vi "IP to Equipment.vi"(0 "RLT Equipment In":T2={"COM A"="COM3", "MW100"="MW100", "AG34970"="A-34972A", "COM B"="COM4", "COM C"="COM5", "COM D"="COM6"}, 2 "MW100 Semiphore":T3, 5 "Equipment In":T1={"COM Port"="COM3", "MW100"="MW100", "AG34970"="A-34972A", "Chamber"="WT500"}, 7 "Enable":bool, 11 "Error In":errorcluster) -> (4 "RLT Equip Out":T2, 6 "Equipment Out":T1={"COM Port"="COM3", "MW100"="MW100", "AG34970"="A-34972A", "Chamber"="WT500"}, 15 "Error Out":errorcluster)   [LabVIEW 2012]
uses:
  EquipReferences.ctl
  <vilib>/Utility/config.llb/Read Key (String).vi
  <vilib>/Utility/config.llb/Write Key (String).vi
  <vilib>/Utility/config.llb/NI_LVConfig.lvlib
panel:
  out "States":string[](array[string])
  in  "OK":bool
  in  "configuration file path":path=path "C:/work/flowconfig.ini"
  out "read buffer":string
  out "Error History":string[](array[string])
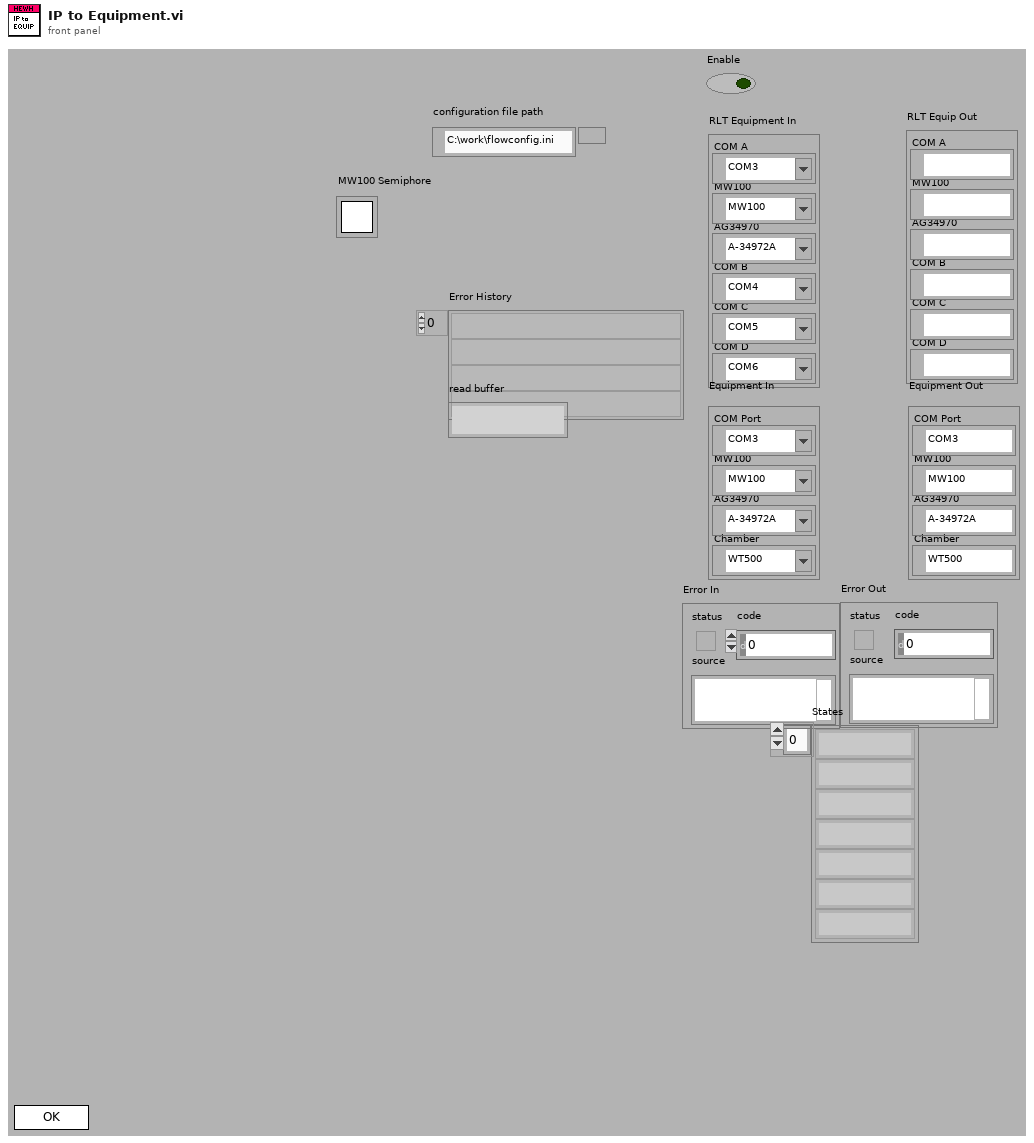
[diagram p1: front panel]
types:
  T1 = typedef "EquipReferences.ctl" = cluster{"COM Port":refnum<visa-resource-name>, "MW100":refnum<visa-resource-name>, "AG34970":refnum<visa-resource-name>, "Chamber":refnum<visa-resource-name>}
  T2 = cluster{"COM A":refnum<visa-resource-name>, "MW100":refnum<visa-resource-name>, "AG34970":refnum<visa-resource-name>, "COM B":refnum<visa-resource-name>, "COM C":refnum<visa-resource-name>, "COM D":refnum<visa-resource-name>}
  T3 = typedef "Semaphore RefNum" = refnum<k1>
  T4 = enum32{"invalid app kind", "Development System", "Run Time System", "Student Edition", "Embedded LabVIEW", "Evaluation", "Custom"}
  T5 = enum32{"Invalid", "Standard", "Closed", "Hidden", "Minimized", "Maximized"}
  T6 = cluster{"Core":cluster{"Current VI Reference":refnum<vi>, "Close Panel on Exit?":bool}, "Equipment In":T1, "RLT Equipment In":cluster{"COM A":refnum<visa-resource-name>, "MW100":refnum<visa-resource-name>, "AG34970":refnum<visa-resource-name>, "COM B":refnum<visa-resource-name>, "COM C":refnum<visa-resource-name>, "COM D":refnum<visa-resource-name>}, "configuration file path":path, "Error Flag":bool, "IP MW100":string, "IP A34972A":string, "semaphore":T3, "Local?":bool}
  T7 = cluster{"Current VI Reference":refnum<vi>, "Close Panel on Exit?":bool}
  T8 = typedef "NI_LVConfig.lvlib/Config Data RefNum.ctl" = refnum<k1>
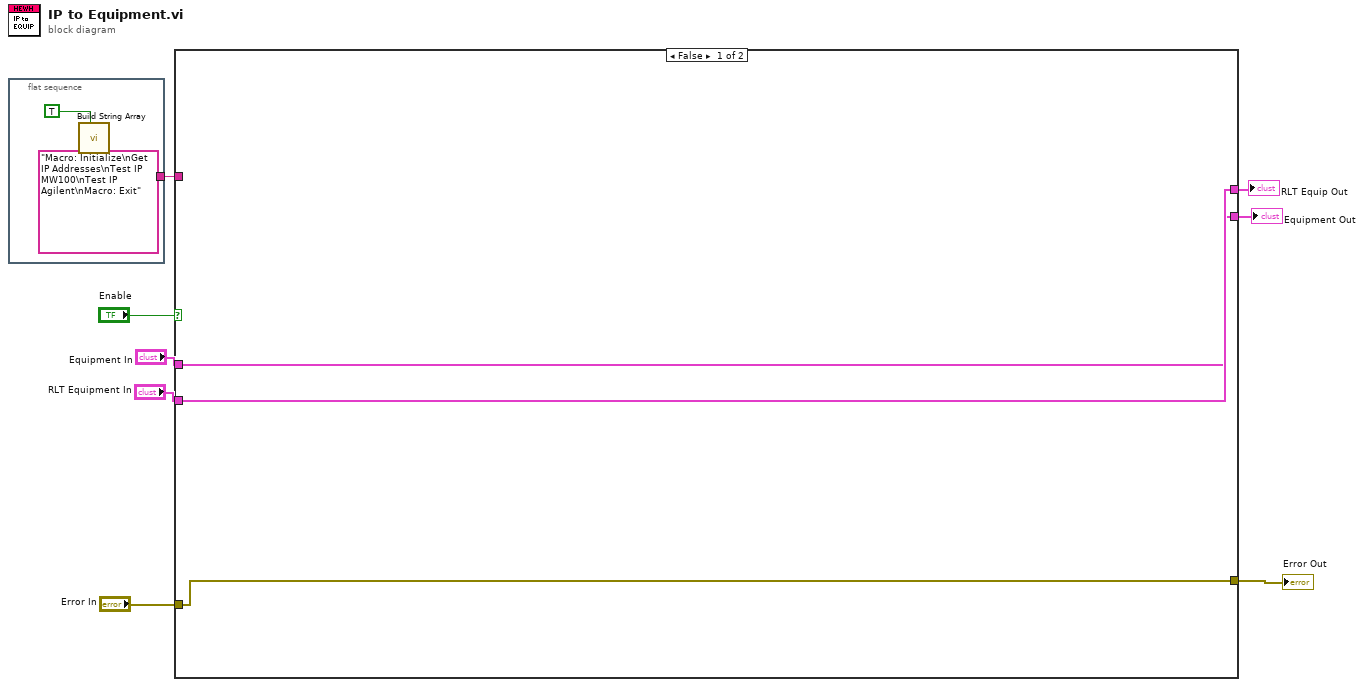
[diagram p0: block diagram]
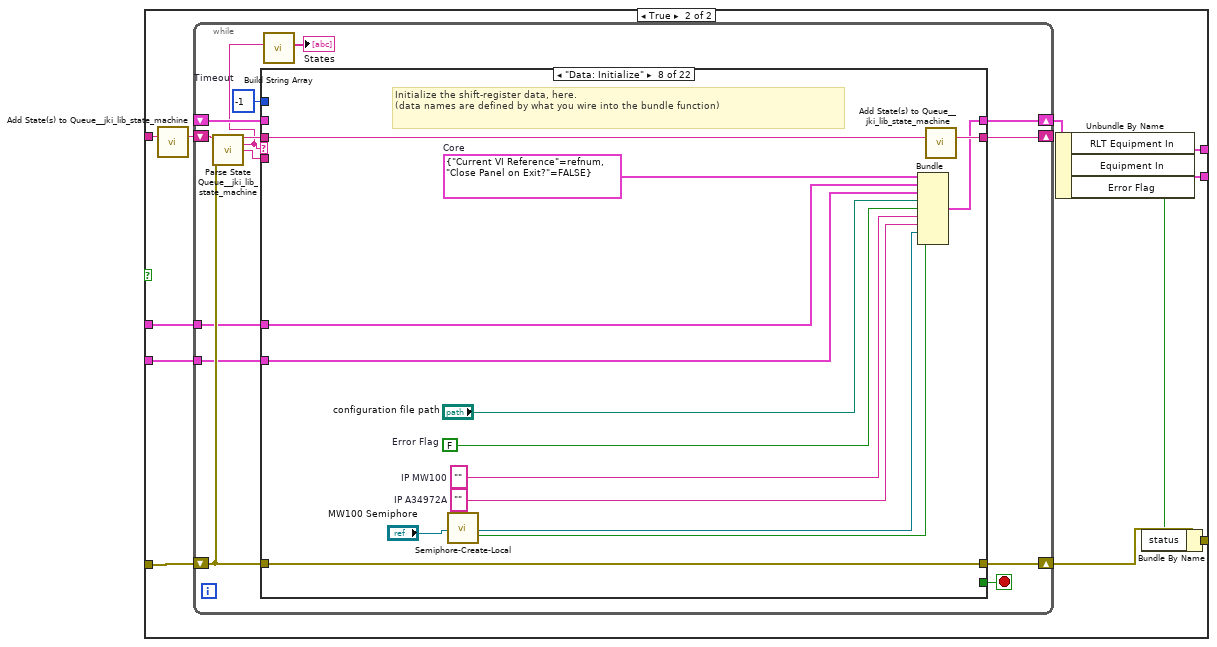
[diagram p2: hidden frame]
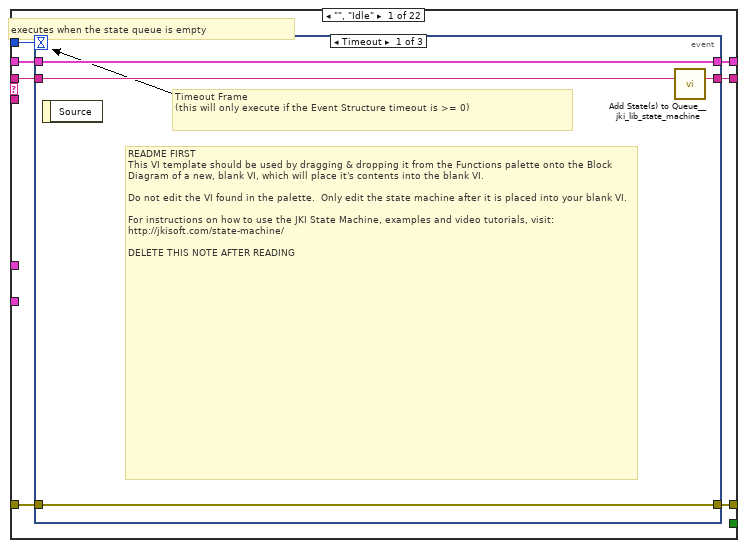
[diagram p3: hidden frame]
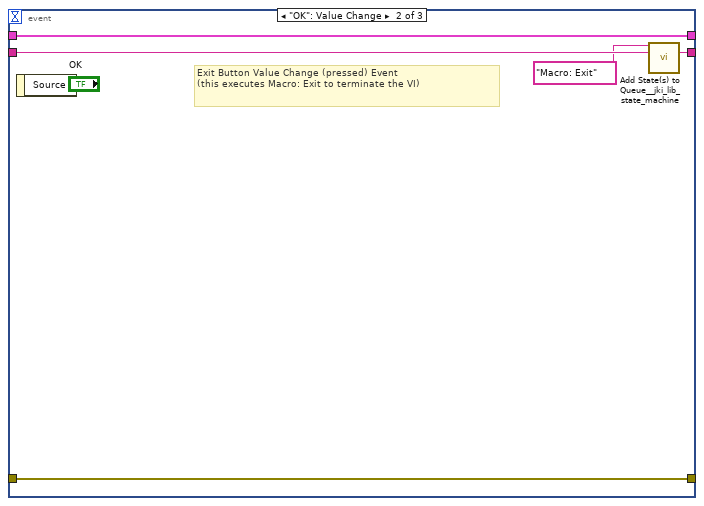
[diagram p4: hidden frame]
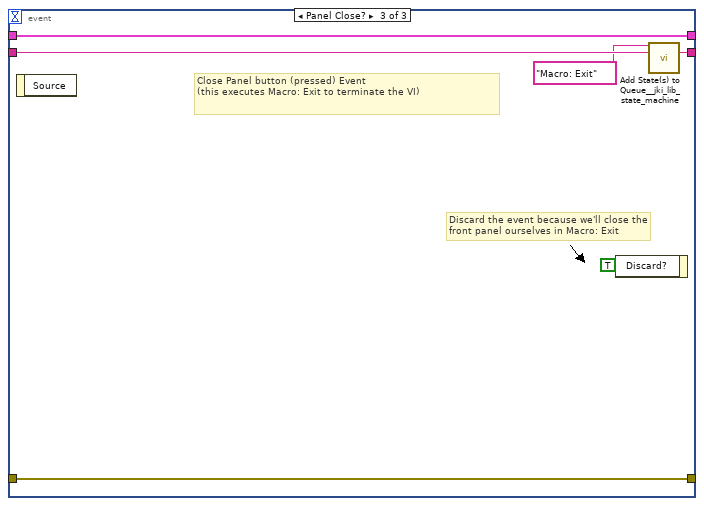
[diagram p5: hidden frame]
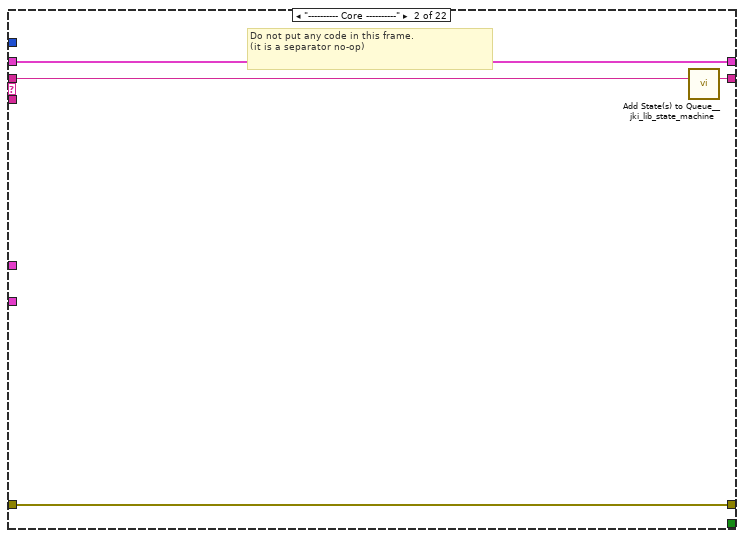
[diagram p6: hidden frame]
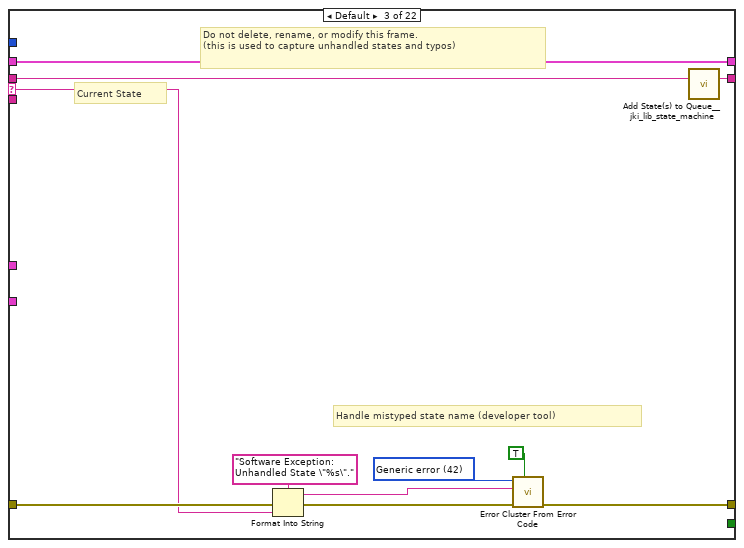
[diagram p7: hidden frame]
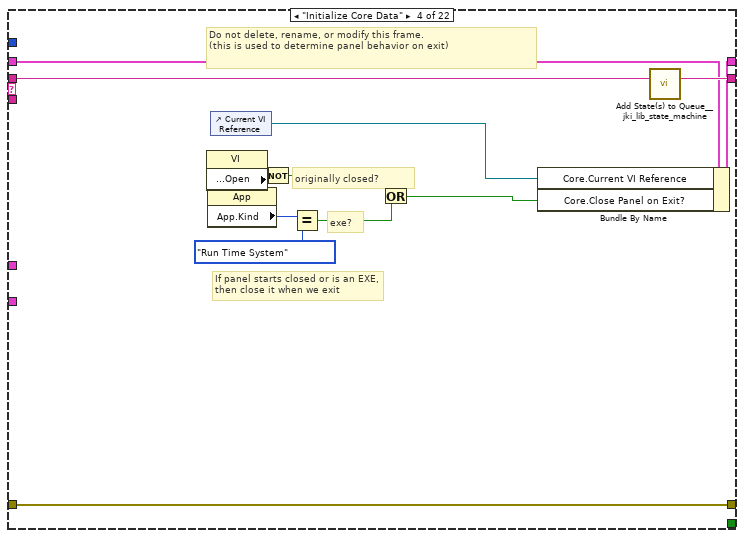
[diagram p8: hidden frame]
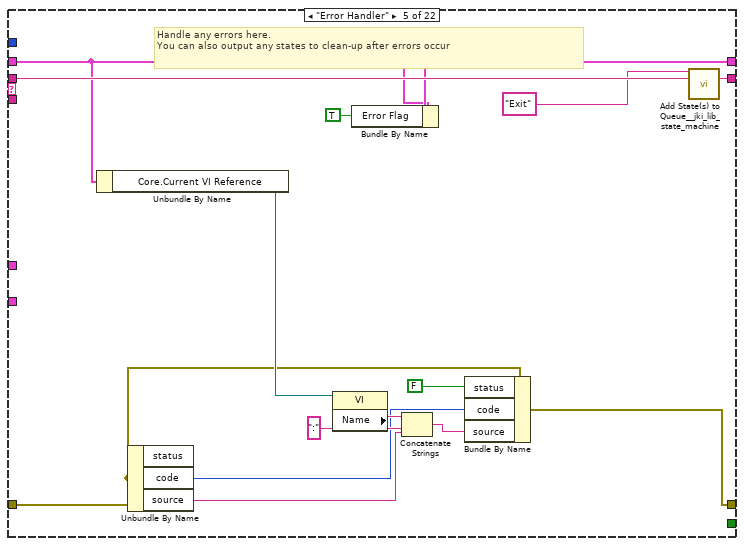
[diagram p9: hidden frame]
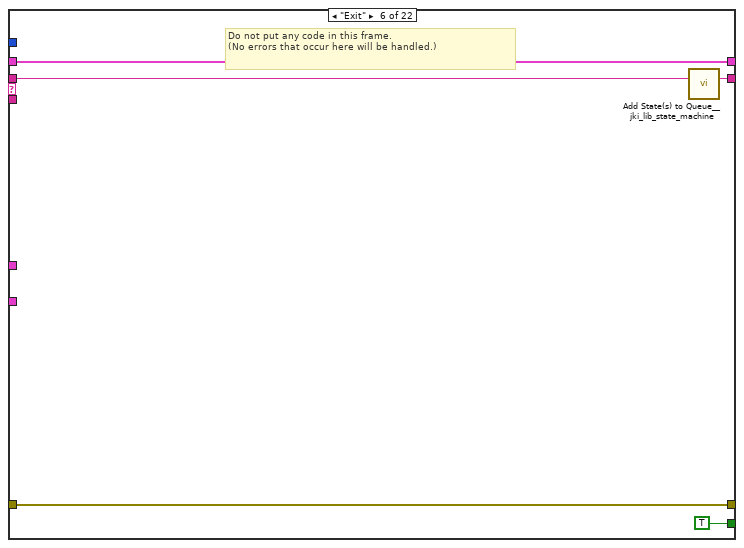
[diagram p10: hidden frame]
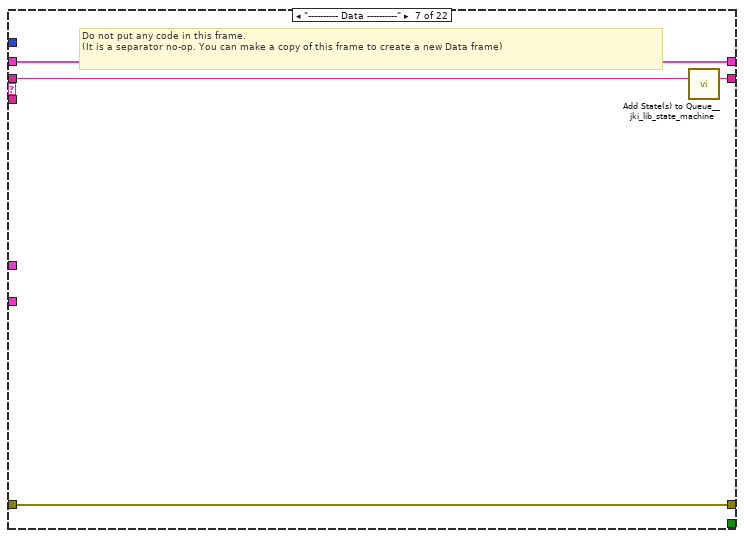
[diagram p11: hidden frame]
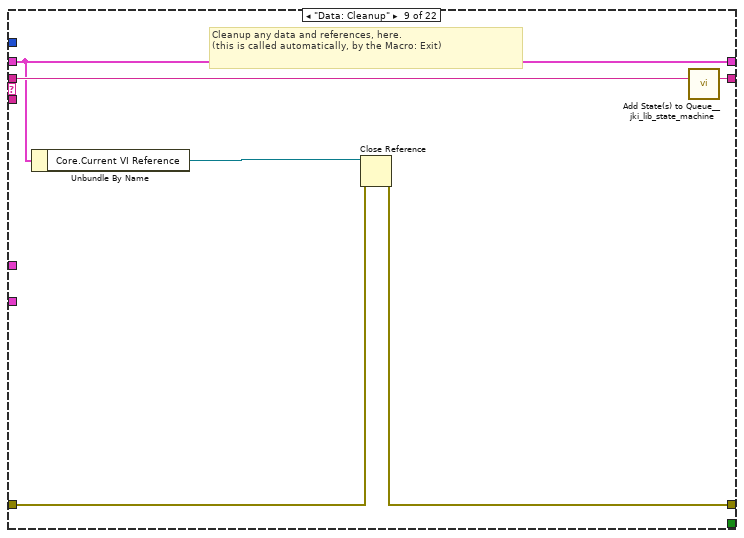
[diagram p12: hidden frame]
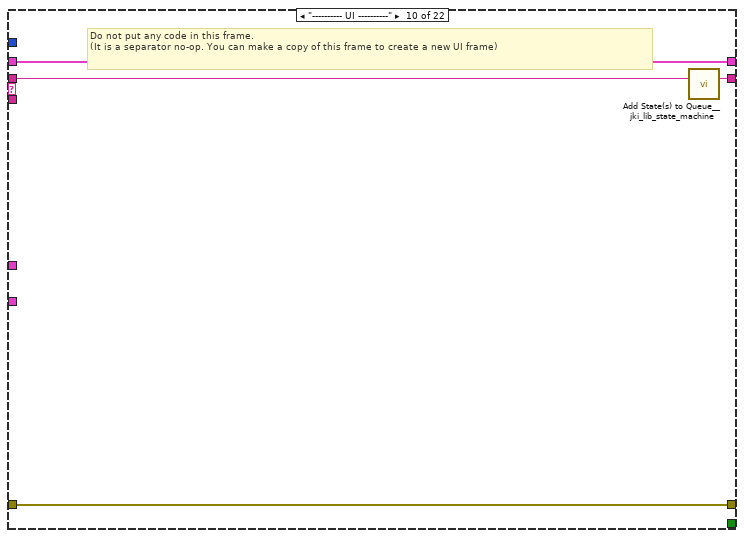
[diagram p13: hidden frame]
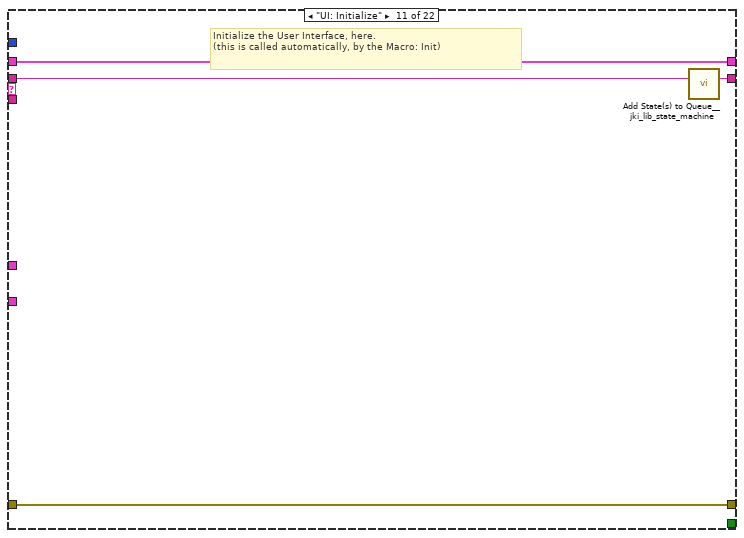
[diagram p14: hidden frame]
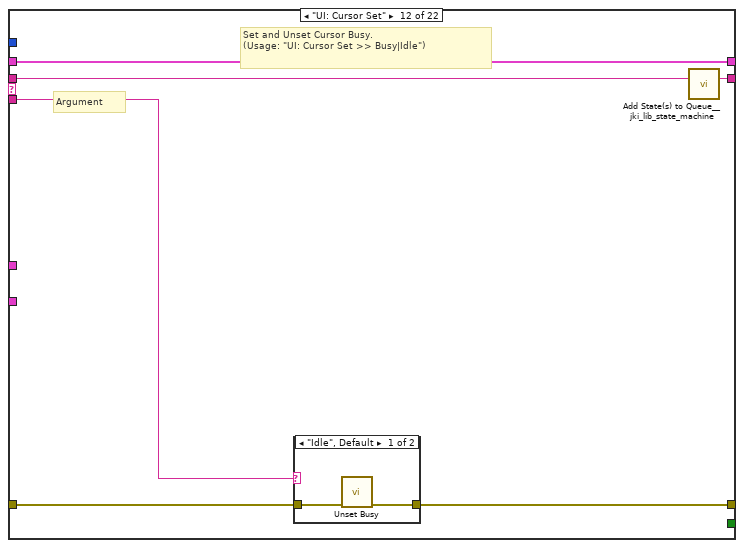
[diagram p15: hidden frame]
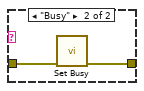
[diagram p16: hidden frame]
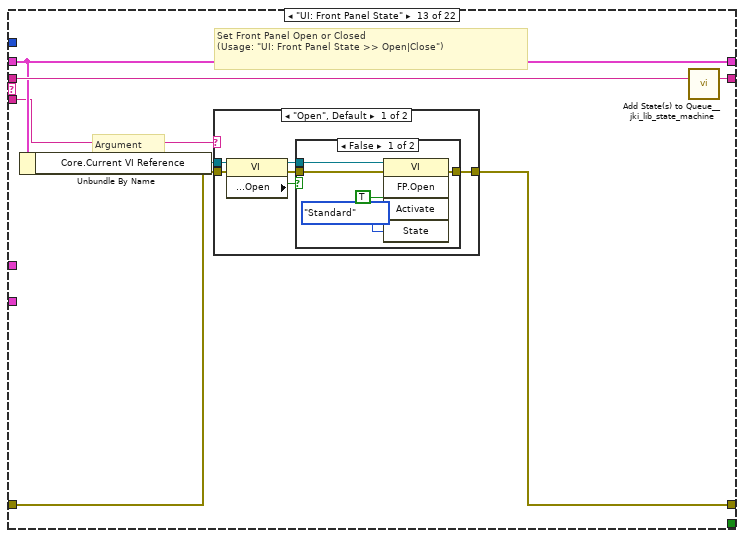
[diagram p17: hidden frame]
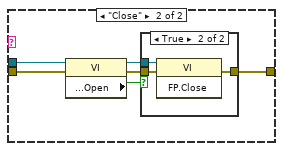
[diagram p19: hidden frame]
diagram:
  n1 = flat-sequence {
    tunnel: ["Macro: Initialize\nGet IP Addresses\nTest IP MW100\nTest IP Agilent\nMacro: Exit"] -> w8
    frame #0 {
      n2 = call "Build String Array.vi"("Initialize"=TRUE) -> ()  [unwired: 10 in, 1 out]
    }
  }
  n3 = case shown="False" "Enable" {
    tunnel: w8 -> [_ w23]
    tunnel: "Error In" -> [w11 w22]
    tunnel: [w11 w20] -> w6
    tunnel: [w13 w17] -> w5
    tunnel: [w12 w16] -> w4
    tunnel: "Equipment In" -> [w12 w15]
    tunnel: "RLT Equipment In" -> [w13 w14]
    frame False {
    }
    frame True {
      n4 = call <vilib>:"Add State(s) to Queue__jki_lib_state_machine.vi"("State(s) in (\"\")"=w23) -> ("States Out"=w24:string)  [unwired: 14 in]
      n5 = while {
        shift-right: [w32] -> w21
        shift-left: _ -> [w31]
        shift-right: [w35] -> w19
        shift-left: w22 -> [w29]
        shift-right: [w34] -> _
        shift-left: w24 -> [w36]
        tunnel: w15 -> [w26]
        tunnel: w14 -> [w25]
        stop <- w33 stop-if-true
        w30 = -1  # Timeout
        n6 = call <vilib>:"Parse State Queue__jki_lib_state_machine.vi"("State Queue"=w36, "Error In (no error)"=w29) -> ("Remaining States"=w38:string, "Current State"=w27:string, "Arguments"=w37:string)  [unwired: 11 in]
        n7 = case shown="\"Data: Initialize\"" w27 {
          selector: w27 -> [_ _ w65 _ _ _ _ _ _ _ _ _ _ _ _ _ _ _ _ _ _ _]
          tunnel: w38 -> [w45 w64 w69 w87 w102 w107 w111 w125 w131 w135 w139 w145 w156 w182 w187 w200 w204 w227 w238 w259 w272 w293]
          tunnel: w37 -> [_ _ _ _ _ _ _ _ _ _ _ w140 w150 _ _ _ _ _ _ _ _ _]
          tunnel: w31 -> [w43 w61 w67 w78 w93 w103 w108 _ w126 w132 w137 w143 w152 w179 w184 w190 w201 w215 w235 w242 w262 w287]
          tunnel: [w42 w62 w71 w84 w89 w105 w109 w122 w127 w133 w136 w141 w153 w180 w185 w188 w202 w205 w236 w246 w270 w291] -> w35
          tunnel: w29 -> [w41 w62 w70 w84 w88 w105 w109 w122 w128 w133 w136 w142 w154 w180 w185 w189 w202 w220 w236 w256 w270 w291]
          tunnel: [w44 w63 w68 w86 w101 w106 w110 w124 w130 w134 w138 w144 w155 w181 w186 w199 w203 w226 w237 w258 w271 w292] -> w34
          tunnel: [_ _ _ _ _ TRUE _ _ _ _ _ _ _ _ _ _ _ _ _ _ _ _] -> w33
          tunnel: [w40 w61 w67 w85 w99 w103 w108 w123 w126 w132 w137 w143 w152 w179 w184 w190 w201 w214 w235 w243 w261 w286] -> w32
          tunnel: w30 -> [w39 _ _ _ _ _ _ _ _ _ _ _ _ _ _ _ _ _ _ _ _ _]
          tunnel: w26 -> [_ _ _ _ _ _ _ w113 _ _ _ _ _ _ _ _ _ _ _ _ _ _]
          tunnel: w25 -> [_ _ _ _ _ _ _ w112 _ _ _ _ _ _ _ _ _ _ _ _ _ _]
          frame "", "Idle" {
            # "executes when the state queue is empty"
            n8 = event shown="[0] Timeout" {
              selector: _ -> [_ _ _]
              dyn-events: _ -> [_ _ _]
              timeout: w39 -> [_ _ _]
              tunnel: w45 -> [w49 w54 w60]
              tunnel: [w48 w53 w59] -> w44
              tunnel: w43 -> [w46 w51 w57]
              tunnel: [w47 w52 w58] -> w42
              tunnel: w41 -> [w47 w52 w58]
              tunnel: [w46 w51 w57] -> w40
              event Timeout {
                # "README FIRST\nThis VI template should be used by dragging & dropping it from the Functions palette onto the Block Diagram of a new, blank VI, which will place it's contents into the blank VI.\n\nDo not edit the VI found in the palette.  Only edit the state machine after it is placed into your blank VI.\n\nFor instructions on how to use the JKI State Machine, examples and video tutorials, visit:\nhttp://jkisoft.com/state-machine/\n\nDELETE THIS NOTE AFTER READING"
                # "Timeout Frame\n(this will only execute if the Event Structure timeout is >= 0)"
                n9 = event-data() -> ()  [unwired: 1 in, 1 out]
                n10 = call <vilib>:"Add State(s) to Queue__jki_lib_state_machine.vi"("State(s) in (\"\")"=w49) -> ("States Out"=w48:string)  [unwired: 14 in]
              }
              event "OK": Value Change {
                # "Exit Button Value Change (pressed) Event\n(this executes Macro: Exit to terminate the VI)"
                n11 = event-data() -> ()  [unwired: 1 in, 1 out]
                n12 = call <vilib>:"Add State(s) to Queue__jki_lib_state_machine.vi"("State(s) in Front (\"\")"="Macro: Exit", "State(s) in (\"\")"=w54) -> ("States Out"=w53:string)  [unwired: 13 in]
              }
              event Panel Close? {
                # "Discard the event because we'll close the front panel ourselves in Macro: Exit"
                # "Close Panel button (pressed) Event\n(this executes Macro: Exit to terminate the VI)"
                n13 = event-data() -> ()  [unwired: 1 in, 1 out]
                n14 = event-data("Discard?"=TRUE) -> ()  [unwired: 1 in, 1 out]
                n15 = call <vilib>:"Add State(s) to Queue__jki_lib_state_machine.vi"("State(s) in Front (\"\")"="Macro: Exit", "State(s) in (\"\")"=w60) -> ("States Out"=w59:string)  [unwired: 13 in]
              }
            }
          }
          frame "---------- Core ----------" {
            # "Do not put any code in this frame.\n(it is a separator no-op)"
            n16 = call <vilib>:"Add State(s) to Queue__jki_lib_state_machine.vi"("State(s) in (\"\")"=w64) -> ("States Out"=w63:string)  [unwired: 14 in]
          }
          frame Default {
            w74 = 42 items=["No error", "Argument error", "Memory is full", "Out of zone", "End of file", "File already open", "Generic file I/O error", "File not found", "File permission error", "Disk is full", "Duplicate path", "Too many files open", "System feature not enabled", "Resource file not found", "Cannot add resource", "Resource not found", "Image not found", "Image memory error", "Pen does not exist", "Config type invalid", "Config token not found", "Config parse error", "Config memory error", "Bad external code format", "Bad external code offset", "External code not present", "Null window", "Destroy window error", "Null menu", "Print aborted", "Bad print record", "Print driver error", "Windows error during printing", "Memory error during printing", "Print dialog error", "Generic print error", "Invalid device refnum", "Device not found", "Device parameter error", "Device unit error", "Cannot open device", "Device call aborted", "Generic error", "Cancelled by user", "Object ID too low", "Object ID too high", "Object not in heap", "Unknown heap", "Unknown object (invalid DefProc)", "Unknown object (DefProc not in table)", "Message out of range", "Invalid (null) method", "Unknown message", "Manager call not supported", "Bad address", "Network operation in progress", "Network operation timed out", "Connection is busy", "Network attribute not supported", "Network error", "Address in use", "System out of memory", "Connection aborted", "Connection refused", "Not connected", "Already connected", "Connection closed", "Initialization error (interapplication manager)", "Bad occurrence", "Wait on unbound occurrence handler", "Occurrence queue overflow", "Datalog type conflict", "Unused", "Unrecognized type (interapplication manager)", "Memory corrupt", "Failed to make temporary DLL", "Old CIN version", "Drag socket not found", "Failed to load drop-object", "Failed to register OLE object", "Failed to release OLE object", "Format specifier type mismatch", "Unknown format specifier", "Too few format specifiers", "Too many format specifiers", "Scan failed", "Newer CIN version", "Error converting to variant", "Runtime menu error", "Password tampered", "Variant attribute not found", "Incompatible variant data type", "Event data is not available", "Event Store is not present", "Occurrence is not found", "Event Queue is not created", "Event info is not available", "Refnum passed is NULL", "Error retrieving Class GUID", "Error retrieving CoClass GUID", "Error retrieving TypeLib GUID.", "Bad built application magic bytes.", "Specific driver is different from the specific driver associated with the Logical Name.", "There is no session opened to the class driver.", "Max Error", "MAX - Error with config objects", "MAX - Error loading configuration", "MAX - Group not supported"]
            # "Current State"
            # "Do not delete, rename, or modify this frame.\n(this is used to capture unhandled states and typos)"
            # "Handle mistyped state name (developer tool)"
            n17 = Format Into String(format string="Software Exception: Unhandled State \"%s\"." ("message"), error in=w70, w65) -> (resulting string=w73:string, error out=w72:errorcluster)  [unwired: 1 in]
            n18 = call <vilib>:"Error Cluster From Error Code.vi"("show call chain? (False)"=TRUE, "error in (no error)"=w72, "error message (\"\")"=w73, "error code (0)"=w74) -> ("error out"=w71:errorcluster)  [unwired: 5 in]
            n19 = call <vilib>:"Add State(s) to Queue__jki_lib_state_machine.vi"("State(s) in (\"\")"=w69) -> ("States Out"=w68:string)  [unwired: 14 in]
          }
          frame "Initialize Core Data" {
            # "Do not delete, rename, or modify this frame.\n(this is used to determine panel behavior on exit)"
            # "originally closed?"
            # "exe?"
            # "If panel starts closed or is an EXE, then close it when we exit"
            n20 = property class="VI"() -> ("Front Panel.Open"=w83:bool)  [unwired: 2 in, 2 out]
            n21 = property class="App"() -> ("App.Kind"=w82:T4)  [unwired: 2 in, 2 out]
            n22 = control-ref of="Current VI Reference"() -> (w76:refnum<vi>)
            n23 = Not(x=w83) -> (.not. x?=w80:bool)
            n24 = Equal?(x=w82, y=T4."Run Time System" ("Application:Kind")) -> (x = y?=w79:bool)
            n25 = Or(x=w80, y=w79) -> (x .or. y?=w77:bool)
            n26 = Bundle By Name(cluster=w78, "Core.Current VI Reference"=w76, "Core.Close Panel on Exit?"=w77) -> (w85:T6)
            n27 = call <vilib>:"Add State(s) to Queue__jki_lib_state_machine.vi"("State(s) in (\"\")"=w87) -> ("States Out"=w86:string)  [unwired: 14 in]
          }
          frame "Error Handler" {
            # "Handle any errors here.\nYou can also output any states to clean-up after errors occur"
            n28 = Unbundle By Name(w93) -> ("Core.Current VI Reference"=w92:refnum<vi>)
            n29 = Unbundle By Name(w88) -> ("code"=w91:i32, "source"=w90:string)  [unwired: 1 out]
            n30 = property class="VI"(reference=w92) -> ("Name"=w94:string)  [unwired: 1 in, 2 out]
            n31 = Bundle By Name(cluster=w93, "Error Flag"=TRUE) -> (w99:T6)
            n32 = Concatenate Strings(w94, ":" ("string"), w90) -> (w96:string)
            n33 = Bundle By Name(cluster=w88, "status"=FALSE, "code"=w91, "source"=w96) -> (w89:errorcluster)
            n34 = call <vilib>:"Add State(s) to Queue__jki_lib_state_machine.vi"("State(s) in Front (\"\")"="Exit", "State(s) in (\"\")"=w102) -> ("States Out"=w101:string)  [unwired: 13 in]
          }
          frame "Exit" {
            # "Do not put any code in this frame.\n(No errors that occur here will be handled.)"
            n35 = call <vilib>:"Add State(s) to Queue__jki_lib_state_machine.vi"("State(s) in (\"\")"=w107) -> ("States Out"=w106:string)  [unwired: 14 in]
          }
          frame "---------- Data ----------" {
            # "Do not put any code in this frame.\n(It is a separator no-op. You can make a copy of this frame to create a new Data frame)"
            n36 = call <vilib>:"Add State(s) to Queue__jki_lib_state_machine.vi"("State(s) in (\"\")"=w111) -> ("States Out"=w110:string)  [unwired: 14 in]
          }
          frame "Data: Initialize" {
            w116 = ""  # IP A34972A
            w117 = ""  # IP MW100
            w118 = FALSE  # Error Flag
            w121 = T7 {"Current VI Reference"=refnum, "Close Panel on Exit?"=FALSE}  # Core
            # "Initialize the shift-register data, here.\n(data names are defined by what you wire into the bundle function)"
            n37 = call "Semiphore-Create-Local.vi"("Semiphore"="MW100 Semiphore") -> ("semaphore"=w115:T3, "Local?"=w114:bool)  [unwired: 16 in, 1 out]
            n38 = Bundle("Core"=w121, "Equipment In"=w113, "RLT Equipment In"=w112, "configuration file path"="configuration file path", "Error Flag"=w118, "IP MW100"=w117, "IP A34972A"=w116, "semaphore"=w115, "Local?"=w114) -> (w123:T6)  [unwired: 1 in]
            n39 = call <vilib>:"Add State(s) to Queue__jki_lib_state_machine.vi"("State(s) in (\"\")"=w125) -> ("States Out"=w124:string)  [unwired: 14 in]
          }
          frame "Data: Cleanup" {
            # "Cleanup any data and references, here.\n(this is called automatically, by the Macro: Exit)"
            n40 = Unbundle By Name(w126) -> ("Core.Current VI Reference"=w129:refnum<vi>)
            n41 = Close Reference(reference=w129, error in (no error)=w128) -> (error out=w127:errorcluster)
            n42 = call <vilib>:"Add State(s) to Queue__jki_lib_state_machine.vi"("State(s) in (\"\")"=w131) -> ("States Out"=w130:string)  [unwired: 14 in]
          }
          frame "---------- UI ----------" {
            # "Do not put any code in this frame.\n(It is a separator no-op. You can make a copy of this frame to create a new UI frame)"
            n43 = call <vilib>:"Add State(s) to Queue__jki_lib_state_machine.vi"("State(s) in (\"\")"=w135) -> ("States Out"=w134:string)  [unwired: 14 in]
          }
          frame "UI: Initialize" {
            # "Initialize the User Interface, here.\n(this is called automatically, by the Macro: Init)"
            n44 = call <vilib>:"Add State(s) to Queue__jki_lib_state_machine.vi"("State(s) in (\"\")"=w139) -> ("States Out"=w138:string)  [unwired: 14 in]
          }
          frame "UI: Cursor Set" {
            # "Argument"
            # "Set and Unset Cursor Busy.\n(Usage: \"UI: Cursor Set >> Busy|Idle\")"
            n45 = case shown="\"Idle\", Default" w140 {
              tunnel: w142 -> [w147 w149]
              tunnel: [w146 w148] -> w141
              frame "Idle", Default {
                n46 = call <vilib>:"Unset Busy.vi"("error in (no error)"=w147) -> ("error out"=w146:errorcluster)  [unwired: 10 in]
              }
              frame "Busy" {
                n47 = call <vilib>:"Set Busy.vi"("error in (no error)"=w149) -> ("error out"=w148:errorcluster)  [unwired: 9 in, 1 out]
              }
            }
            n48 = call <vilib>:"Add State(s) to Queue__jki_lib_state_machine.vi"("State(s) in (\"\")"=w145) -> ("States Out"=w144:string)  [unwired: 14 in]
          }
          frame "UI: Front Panel State" {
            # "Argument"
            # "Set Front Panel Open or Closed\n(Usage: \"UI: Front Panel State >> Open|Close\")"
            n49 = Unbundle By Name(w152) -> ("Core.Current VI Reference"=w151:refnum<vi>)
            n50 = case shown="\"Open\", Default" w150 {
              tunnel: w154 -> [w160 w173]
              tunnel: [w162 w174] -> w153
              tunnel: w151 -> [w161 w171]
              frame "Open", Default {
                n51 = property class="VI"(reference=w161, error in=w160) -> (reference out=w158:refnum<vi>, error out=w159:errorcluster, "Front Panel.Open"=w157:bool)
                n52 = case shown="False" w157 {
                  tunnel: [w165 w168] -> w162
                  tunnel: w159 -> [w164 w168]
                  tunnel: w158 -> [w163 _]
                  frame False {
                    n53 = invoke class="VI" method="FP.Open"(reference=w163, error in=w164, "Activate"=TRUE, "State"=T5."Standard") -> (error out=w165:errorcluster)  [unwired: 1 in, 4 out]
                  }
                  frame True {
                  }
                }
              }
              frame "Close" {
                n54 = property class="VI"(reference=w171, error in=w173) -> (reference out=w170:refnum<vi>, error out=w172:errorcluster, "Front Panel.Open"=w169:bool)
                n55 = case shown="True" w169 {
                  tunnel: [w175 w178] -> w174
                  tunnel: w172 -> [w175 w177]
                  tunnel: w170 -> [_ w176]
                  frame False {
                  }
                  frame True {
                    n56 = invoke class="VI" method="FP.Close"(reference=w176, error in=w177) -> (error out=w178:errorcluster)  [unwired: 1 in, 2 out]
                  }
                }
              }
            }
            n57 = call <vilib>:"Add State(s) to Queue__jki_lib_state_machine.vi"("State(s) in (\"\")"=w156) -> ("States Out"=w155:string)  [unwired: 14 in]
          }
          frame "---------- Macro ----------" {
            # "Do not put any code in this frame.\n(It is a separator no-op. You can make a copy of this frame to create a new Macro frame)"
            n58 = call <vilib>:"Add State(s) to Queue__jki_lib_state_machine.vi"("State(s) in (\"\")"=w182) -> ("States Out"=w181:string)  [unwired: 14 in]
          }
          frame "Macro: Initialize" {
            # "Initialization Macro\n(This is called once, when the VI starts)"
            n59 = call <vilib>:"Add State(s) to Queue__jki_lib_state_machine.vi"("State(s) in Front (\"\")"="Data: Initialize\nInitialize Core Data", "State(s) in (\"\")"=w187) -> ("States Out"=w186:string)  [unwired: 13 in]
          }
          frame "Macro: Exit" {
            # "Exit Macro\n(This is called once, when the VI exits)"
            n60 = Unbundle By Name(w190) -> ("Core.Close Panel on Exit?"=w198:bool)
            n61 = Unbundle By Name(w190) -> ("semaphore"=w192:T3, "Local?"=w191:bool)
            n62 = call "Semiphore-Destroy-Local.vi"("Semiphore"=w192, "Local?"=w191, "error in (no error)"=w189) -> ("error out"=w188:errorcluster)  [unwired: 16 in]
            n63 = Select(t="UI: Front Panel State >> Close", s=w198, f="") -> (s? t:f=w195:string)
            n64 = call <vilib>:"Add State(s) to Queue__jki_lib_state_machine.vi"("State(s) in (\"\")"=w195, "State(s) at Back (\"\")"="Data: Cleanup\nExit") -> ("States Out"=w193:string)  [unwired: 13 in]
            n65 = call <vilib>:"Add State(s) to Queue__jki_lib_state_machine.vi"("State(s) in Front (\"\")"=w193, "State(s) in (\"\")"=w200) -> ("States Out"=w199:string)  [unwired: 13 in]
          }
          frame "---------- New Category ----------" {
            # "Template Separator\n(You can make a copy of, or modify, this frame)"
            n66 = call <vilib>:"Add State(s) to Queue__jki_lib_state_machine.vi"("State(s) in (\"\")"=w204) -> ("States Out"=w203:string)  [unwired: 14 in]
          }
          frame "Get IP Addresses" {
            w222 = "IP Addresses" ("section")
            n67 = Unbundle By Name(w215) -> ("configuration file path"=w218:path)
            n68 = call <vilib>:"Open Config Data.vi"("error in (no error)"=w220, "create file if necessary (T)"=FALSE, "configuration file path"=w218) -> ("error out"=w221:errorcluster, "refnum"=w223:T8)  [unwired: 6 in, 1 out]
            n69 = call-poly <vilib>:"Read Key.vi"("section"=w222, "error in (no error)"=w221, "key"="IP MW100", "refnum"=w223) -> ("error out"=w225:errorcluster, "value"=w213:string, "found?"=w209:bool, "refnum out"=w224:T8)  [unwired: 4 in]
            n70 = call-poly <vilib>:"Read Key.vi"("section"=w222, "error in (no error)"=w225, "key"="IP A34972A", "refnum"=w224) -> ("error out"=w206:errorcluster, "value"=w212:string, "found?"=w210:bool, "refnum out"=w207:T8)  [unwired: 4 in]
            n71 = call <vilib>:"Close Config Data.vi"("error in (no error)"=w206, "refnum"=w207) -> ("error out"=w205:errorcluster)  [unwired: 8 in, 1 out]
            n72 = And(x=w210, y=w209) -> (x .and. y?=w211:bool)
            n73 = case shown="True" w211 {
              tunnel: w215 -> [w229 w234]
              tunnel: [w229 w233] -> w214
              tunnel: w213 -> [_ w232]
              tunnel: w212 -> [_ w231]
              tunnel: ["Prompt for IP" ("State(s) in Front (\"\")") "" ("State(s) in Front (\"\")")] -> w208
              frame False {
              }
              frame True {
                n74 = Bundle By Name(cluster=w234, "IP MW100"=w232, "IP A34972A"=w231) -> (w233:T6)
              }
            }
            n75 = call <vilib>:"Add State(s) to Queue__jki_lib_state_machine.vi"("State(s) in Front (\"\")"=w208, "State(s) in (\"\")"=w227) -> ("States Out"=w226:string)  [unwired: 13 in]
          }
          frame "Merge IP Addresses" {
            n76 = call <vilib>:"Add State(s) to Queue__jki_lib_state_machine.vi"("State(s) in (\"\")"=w238) -> ("States Out"=w237:string)  [unwired: 14 in]
          }
          frame "Prompt for IP" {
            w252 = "IP Addresses" ("section")
            n77 = Unbundle By Name(w242) -> ("configuration file path"=w241:path, "IP MW100"=w240:string, "IP A34972A"=w239:string)
            n78 = call <vilib>:"Open Config Data.vi"("error in (no error)"=w256, "create file if necessary (T)"=FALSE, "configuration file path"=w241) -> ("error out"=w255:errorcluster, "refnum"=w249:T8)  [unwired: 6 in, 1 out]
            n79 = call "Enter IPs.vi"("34972A IP"=w239, "MW100 IP"=w240) -> ("34972A IP Out"=w244:string, "MW100 IP Out"=w245:string)  [unwired: 8 in]
            n80 = call-poly <vilib>:"Write Key.vi"("section"=w252, "error in (no error)"=w255, "value"=w245, "key"="IP MW100", "refnum"=w249) -> ("error out"=w254:errorcluster, "refnum out"=w248:T8)  [unwired: 4 in, 1 out]
            n81 = call-poly <vilib>:"Write Key.vi"("section"=w252, "error in (no error)"=w254, "value"=w244, "key"="IP A34972A", "refnum"=w248) -> ("error out"=w253:errorcluster, "refnum out"=w247:T8)  [unwired: 4 in, 1 out]
            n82 = call <vilib>:"Close Config Data.vi"("error in (no error)"=w253, "refnum"=w247) -> ("error out"=w246:errorcluster)  [unwired: 8 in, 1 out]
            n83 = Bundle By Name(cluster=w242, "IP MW100"=w245, "IP A34972A"=w244) -> (w243:T6)
            n84 = call <vilib>:"Add State(s) to Queue__jki_lib_state_machine.vi"("State(s) in (\"\")"=w259) -> ("States Out"=w258:string)  [unwired: 14 in]
          }
          frame "Test IP MW100" {
            n85 = Unbundle By Name(w262) -> ("semaphore"=w260:T3, "IP MW100"=w267:string)
            n86 = Concatenate Strings("TCPIP::" ("string"), w267, "::34318::SOCKET" ("string")) -> (w263:string)
            n87 = call "YKMW100 Get Error Log.vi"("VISA session"=w263, "Semiphore"=w260) -> ("Error History"=→"Error History":string[], "error out"=w265:errorcluster)  [unwired: 10 in, 2 out]
            n88 = case shown="No Error" w265 {
              selector: w265 -> [_ w279]
              tunnel: ["" ("State(s) in Front (\"\")") "Prompt for IP\nTest IP MW100\n" ("State(s) in Front (\"\")")] -> w264
              tunnel: w262 -> [w275 w277]
              tunnel: w263 -> [w273 _]
              tunnel: [w274 w277] -> w261
              frame No Error {
                n89 = Bundle By Name(cluster=w275, "Equipment In.MW100"=w273, "RLT Equipment In.MW100"=w273) -> (w274:T6)
              }
              frame Error {
                n90 = call <vilib>:"Simple Error Handler.vi"("error in (no error)"=w279) -> ()  [unwired: 4 in, 5 out]
              }
            }
            n91 = call <vilib>:"Add State(s) to Queue__jki_lib_state_machine.vi"("State(s) in Front (\"\")"=w264, "State(s) in (\"\")"=w272) -> ("States Out"=w271:string)  [unwired: 13 in]
          }
          frame "Test IP Agilent" {
            # "::inst0::INSTR"
            n92 = Unbundle By Name(w287) -> ("IP A34972A"=w289:string)  [unwired: 1 out]
            n93 = disable-structure shown="Enabled" {
              disable-tunnel: ["::5025::SOCKET" ("string") "::inst0::INSTR" ("string")] -> w281
              frame Disabled {
              }
              frame Enabled {
              }
            }
            n94 = Concatenate Strings("TCPIP::" ("string"), w289, w281) -> (w280:string)
            n95 = call "Agilent Scan EZ Temperature.vi"("VISA Resource Name"=w280, "Control"=enum16{"Initialize", "Read", "Experiment"}."Initialize", "Channel Input"="101") -> ("read buffer"=→"read buffer":string, "error out"=w283:errorcluster)  [unwired: 9 in, 2 out]
            n96 = case shown="No Error" w283 {
              selector: w283 -> [_ w302]
              tunnel: ["" ("State(s) in Front (\"\")") "Prompt for IP\nTest IP MW100\nTest IP Agilent" ("State(s) in Front (\"\")")] -> w288
              tunnel: w287 -> [w298 w300]
              tunnel: w280 -> [w296 _]
              tunnel: [w297 w300] -> w286
              frame No Error {
                n97 = Bundle By Name(cluster=w298, "Equipment In.AG34970"=w296, "RLT Equipment In.AG34970"=w296) -> (w297:T6)
              }
              frame Error {
                n98 = call <vilib>:"Simple Error Handler.vi"("error in (no error)"=w302) -> ()  [unwired: 4 in, 5 out]
              }
            }
            n99 = call <vilib>:"Add State(s) to Queue__jki_lib_state_machine.vi"("State(s) in Front (\"\")"=w288, "State(s) in (\"\")"=w293) -> ("States Out"=w292:string)  [unwired: 13 in]
          }
        }
        n100 = call "Build String Array.vi"("string"=w27) -> ("Array"=→"States":string[])  [unwired: 10 in]
      }
      n101 = Unbundle By Name(w21) -> ("RLT Equipment In"=w17:T2, "Equipment In"=w16:T1, "Error Flag"=w18:bool)
      n102 = Bundle By Name(cluster=w19, "status"=w18) -> (w20:errorcluster)
    }
  }
  "Error Out" <- w6
  "Equipment Out" <- w4
  "RLT Equip Out" <- w5
